vi "Initialisation_Scanner_Mirror.vi"(5 "error in":errorcluster) -> (19 "error out":errorcluster)   [LabVIEW 2013]
uses:
  Variables/GlobalGetPhysikalInstrumentsOnOff.vi
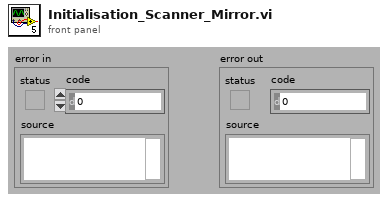
[diagram p1: front panel]
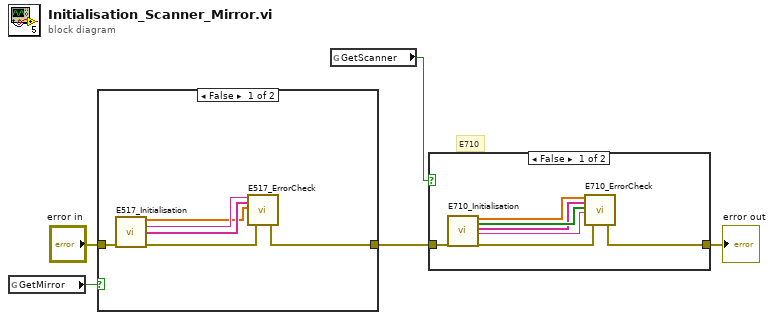
[diagram p0: block diagram]
diagram:
  # "E710"
  n1 = global read "GlobalGetPhysikalInstrumentsOnOff.vi" "GetMirror"() -> (w3:bool)
  n2 = case shown="False" w3 {
    tunnel: [w11 w12] -> w5
    tunnel: "error in" -> [w10 w12]
    frame False {
      n3 = call "E517_Initialisation.vi"("error out"=w10) -> ("Position"=w6:dbl[], "Identification"=w8:string, "Conn. Axes"=w7:string[], "error out 2"=w9:errorcluster)  [unwired: 11 in]
      n4 = call "E517_ErrorCheck.vi"("Identification"=w8, "Conn. Axes"=w7, "Position"=w6, "error out 2"=w9) -> ("error IO"=w11:errorcluster)  [unwired: 15 in]
    }
    frame True {
    }
  }
  n5 = global read "GlobalGetPhysikalInstrumentsOnOff.vi" "GetScanner"() -> (w1:bool)
  n6 = case shown="False" w1 {
    tunnel: [w19 w20] -> w2
    tunnel: w5 -> [w17 w20]
    frame False {
      n7 = call "E710_Initialisation.vi"("error IO"=w17) -> ("Position"=w16:dbl[], "ATZ successful?"=w15:bool[], "Conn. Axes"=w14:string[], "Identification"=w13:string, "error out"=w18:errorcluster)  [unwired: 14 in]
      n8 = call "E710_ErrorCheck.vi"("Position"=w16, "Conn. Axes"=w14, "ATZ successful?"=w15, "Identification"=w13, "error out 2"=w18) -> ("error out"=w19:errorcluster)  [unwired: 14 in]
    }
    frame True {
    }
  }
  "error out" <- w2
